vi "main_VI_one.vi"() -> ()   [LabVIEW 2019]
uses:
  <vilib>/myRIO/Instrument Drivers/Onboard IO/UART/typedef/VISA Configuration.ctl
  <vilib>/Platform/TimedLoop/XDataNode/timing_clust.ctl
  <vilib>/Platform/TimedLoop/XDataNode/nitl_modes.ctl
  <vilib>/Platform/TimedLoop/XDataNode/wakeup.ctl
  <vilib>/Instr/_visa.llb/VISA Configure Serial Port (Instr).vi
  <vilib>/FPGAPlugInAG/myRIO-1900/niLvFpga_Open_myRIO-1900.vi
  <vilib>/rvi/interface/common/dynamic/niFpgaDynamicAddResources.vi
  <vilib>/Utility/error.llb/Error Cluster From Error Code.vi
  <vilib>/rvi/errors/niLvFpgaAdjustHostInterfaceError.vi
  <vilib>/FPGAPlugInAG/Dynamic/niLvFpga_Close_Dynamic.vi
  <vilib>/rvi/interface/nirviOpenFPGA/nirviOpenFPGA.xnode
  FPGA Bitfiles/imuwired_FPGATarget_FPGAFSR_4dEayfvYof8.lvbitx
  <vilib>/Platform/TimedLoop/XDataNode/XDataNode.xnode
  <vilib>/rvi/interface/nirviReadWriteControl/nirviReadWriteControl.xnode
  <vilib>/rvi/interface/nirviCloseFPGA/nirviCloseFPGA.xnode
  <vilib>/Platform/TimedLoop/XDataNode/XDNodeRunTimeDep.lvlib
  <vilib>/myRIO/Instrument Drivers/Onboard IO/UART/UART.lvlib
  NiFpgaLv.dll
  <vilib>/rvi/interface/Simulation/niFpgaSimulationCallBeginRW.vi
panel:
  out "element out 2":dbl
  out "element out":u16
  out "# elements 2":u32
  out "# elements":u32
  out "timed out?":bool
  in  "file no.":u32
  in  "stop":bool
  in  "error in (no error)":errorcluster
  out "error out":errorcluster
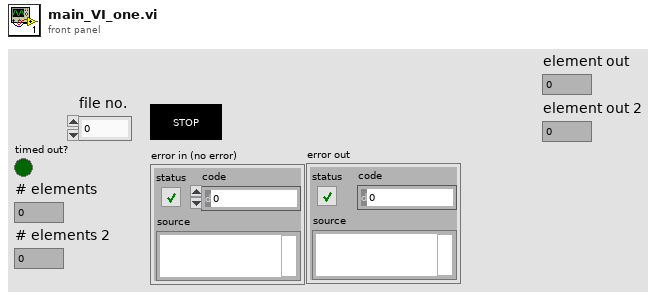
[diagram p1: front panel]
types:
  T1 = enum16{"open", "replace", "create", "open or create", "replace or create", "replace or create with confirmation"}
  T2 = cluster{"read mode":enum16{"polling", "blocking"}, "write mode":enum16{"polling", "blocking"}}
  T3 = typedef "UART.lvlib/VISA Configuration.ctl" = cluster{"baud rate (9600)":u32, "data bits (8)":u16, "parity (0:none)":enum16{"None", "Odd", "Even", "Mark", "Space"}, "stop bits (10: 1 bit)":u16, "flow control (0:none)":u16, "termination char\n(0xA = '\\n' = LF) ":u8, "Enable Termination\nChar (T)":bool, "timeout (10sec)":u32}
  T4 = typedef "XDNodeRunTimeDep.lvlib/timing_clust.ctl" = cluster{"Expected End [f-1]":u64, "Actual End [f-1]":u64, "Finished Late? [f-1]":bool, "Expected End [i-1]":u64, "Actual End [i-1]":u64, "Finished Late? [i-1]":bool, "Expected Start [i]":u64, "Actual Start [i]":u64, "Expected Start [f]":u64, "Actual Start [f]":u64, "Source Name":string, "Structure Name":string, "Period":i64, "Deadline":i64, "Offset":i64, "Start":i64, "Priority":i32, "Timeout":i32, "Mode":T5, "Wakeup Reason":T6, "Error":errorcluster, "Source Type":string, "Secondary Source Type":string, "Global End Time":u64, "Global Start Time":u64, "Frame Duration":u64, "Iteration Duration":u64, "Assigned CPU":i32, "I/O Scan Engine Mode":u32}
  T5 = typedef "XDNodeRunTimeDep.lvlib/nitl_modes.ctl" = enum32{"No Change", "Process missed periods, maintain original phase", "Discard missed periods, maintain original phase", "Process missed periods, ignore original phase", "Discard missed periods, ignore original phase"}
  T6 = typedef "XDNodeRunTimeDep.lvlib/wakeup.ctl" = enum32{"Normal", "Aborted", "Asynchronous wakeup", "Timing source error", "Timed loop error", "Timeout"}
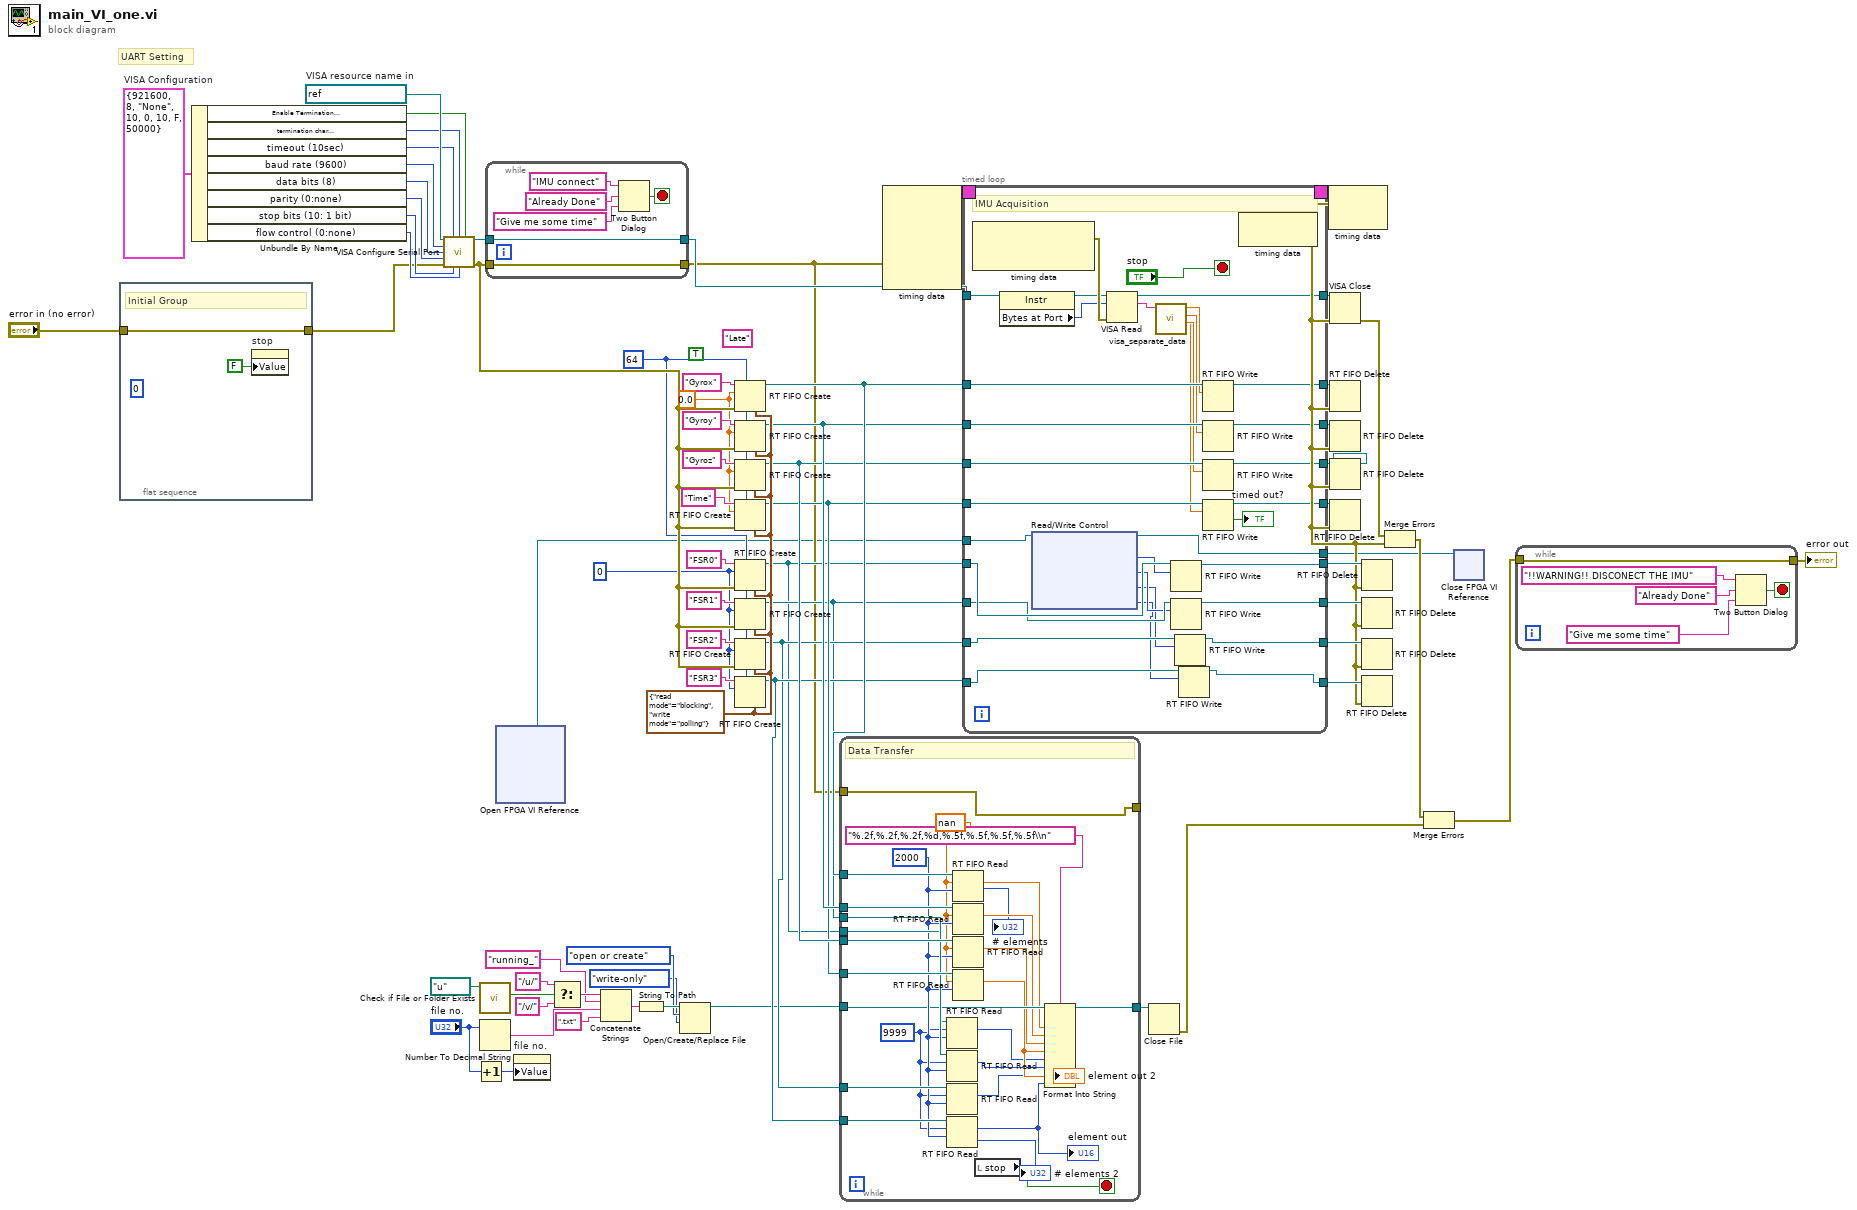
[diagram p0: block diagram]
diagram:
  w2 = u16 0
  w24 = u32 64 ("size (10)")
  (unwired) TRUE
  (unwired) "Late" ("name (unnamed)")
  w47 = T2 {"read mode"=enum."blocking", "write mode"=enum."polling"} ("r/w modes (polling,polling)")
  w25 = 0.0
  w68 = T3 {"baud rate (9600)"=921600, "data bits (8)"=8, "parity (0:none)"=enum."None", "stop bits (10: 1 bit)"=10, "flow control (0:none)"=0, "termination char\n(0xA = '\\n' = LF) "=10, "Enable Termination\nChar (T)"=FALSE, "timeout (10sec)"=50000}  # VISA Configuration
  w69 = refnum<visa-resource-name> "ASRL1::INSTR"  # VISA resource name in
  # "UART Setting"
  n1 = flat-sequence {
    tunnel: "error in (no error)" -> [w73]
    tunnel: [w73] -> w39
    frame #0 {
      (unwired) u16 0 ("On time in")
      # "Initial Group"
      n2 = property on="stop" class="Bool (strict)"("Value"=FALSE ("stop")) -> ()  [unwired: 2 in, 2 out]
    }
  }
  n3 = Unbundle By Name(w68) -> ("Enable Termination\nChar (T)"=w67:bool, "termination char\n(0xA = '\\n' = LF)"=w66:u8, "timeout (10sec)"=w65:u32, "baud rate (9600)"=w61:u32, "data bits (8)"=w62:u16, "parity (0:none)"=w63:enum16{"None", "Odd", "Even", "Mark", "Space"}, "stop bits (10: 1 bit)"=w64:u16, "flow control (0:none)"=w60:u16)
  n4 = call-poly "VISA Configure Serial Port"("VISA resource name"=w69, "timeout (10sec)"=w65, "termination char\n(0xA = '\\n' = LF)"=w66, "Enable Termination\nChar (T)"=w67, "baud rate (9600)"=w61, "data bits (8)"=w62, "parity (0:none)"=w63, "error in (no error)"=w39, "stop bits (10: 1 bit)"=w64, "flow control (0:none)"=w60) -> ("VISA resource name out"=w57:refnum<visa-resource-name>, "error out"=w49:errorcluster)  [unwired: 4 in]
  n5 = Increment(x="file no.") -> (x+1=w11:u32)
  n6 = call <vilib>:"Check if File or Folder Exists.vi"("path"=path "u:/") -> ("file or folder exists?"=w20:bool)  [unwired: 8 in, 2 out]
  n7 = Number To Decimal String(number="file no.") -> (decimal integer string=w14:string)  [unwired: 1 in]
  n8 = while {
    tunnel: [w79] -> w5
    tunnel: w49 -> [w79]
    tunnel: [w78] -> w46
    tunnel: w57 -> [w78]
    stop <- w74 stop-if-true
    n9 = Two Button Dialog(message="IMU connect", 1:"Give me some time" ("F button name (\"Cancel\")"), 2:"Already Done" ("button name (\"OK\")")) -> (T button?=w74:bool)
  }
  n10 = xnode "Open FPGA VI Reference"() -> ("FPGA VI Reference Out"=w3:refnum<k20>)  [unwired: 2 in, 1 out]
  n11 = property on="file no." class="DigNum (strict)"("Value"=w11) -> ()  [unwired: 2 in, 2 out]
  n12 = Select(t="/u/", s=w20, f="/v/") -> (s? t:f=w18:string)
  n13 = Concatenate Strings(w18, "running_" ("string"), w14, ".txt" ("string")) -> (w17:string)
  n14 = String To Path(string=w17) -> (path=w19:path)
  n15 = Open/Create/Replace File(file path (use dialog)=w19, operation (0:open)=T1."open or create", access (0:read/write)=enum16{"read/write", "read-only", "write-only"}."write-only") -> (refnum out=w9:refnum<file>)  [unwired: 3 in, 2 out]
  n16 = RT FIFO Create(0:"Gyrox" ("name (unnamed)"), 1:w25, 3:w49, 4:w24, 7:w47) -> (8:w45:refnum<k33>)  [unwired: 3 in, 2 out]
  n17 = RT FIFO Create(0:"Gyroy" ("name (unnamed)"), 1:w25, 3:w49, 4:w24, 7:w47) -> (8:w44:refnum<k33>)  [unwired: 3 in, 2 out]
  n18 = RT FIFO Create(0:"Gyroz" ("name (unnamed)"), 1:w25, 3:w49, 4:w24, 7:w47) -> (8:w43:refnum<k33>)  [unwired: 3 in, 2 out]
  n19 = RT FIFO Create(0:"Time" ("name (unnamed)"), 1:w25, 3:w49, 4:w24, 7:w47) -> (8:w42:refnum<k33>)  [unwired: 3 in, 2 out]
  n20 = RT FIFO Create(0:"FSR0" ("name (unnamed)"), 1:w2, 3:w49, 4:w24, 7:w47) -> (8:w26:refnum<k33>)  [unwired: 3 in, 2 out]
  n21 = RT FIFO Create(0:"FSR1" ("name (unnamed)"), 1:w2, 3:w49, 4:w24, 7:w47) -> (8:w27:refnum<k33>)  [unwired: 3 in, 2 out]
  n22 = RT FIFO Create(0:"FSR2" ("name (unnamed)"), 1:w2, 3:w49, 4:w24, 7:w47) -> (8:w28:refnum<k33>)  [unwired: 3 in, 2 out]
  n23 = RT FIFO Create(0:"FSR3" ("name (unnamed)"), 1:w2, 4:w24, 7:w47) -> (8:w29:refnum<k33>)  [unwired: 4 in, 2 out]
  n24 = while {
    tunnel: w45 -> [w105]
    tunnel: w44 -> [w104]
    tunnel: w43 -> [w103]
    tunnel: w42 -> [w102]
    tunnel: w29 -> [w101]
    tunnel: w28 -> [w100]
    tunnel: w27 -> [w99]
    tunnel: w26 -> [w98]
    tunnel: w9 -> [w94]
    tunnel: [w84] -> w8
    tunnel: [w95] -> _
    tunnel: w5 -> [w95]
    stop <- w97 stop-if-true
    w80 = u16 9999 ("element")
    w96 = 2000 ("timeout in ms (0)")
    w81 = nan
    # "Data Transfer"
    n25 = RT FIFO Read(0:w98, 1:w80, 2:w96) -> (9:w88:u16)  [unwired: 1 in, 4 out]
    n26 = RT FIFO Read(0:w99, 1:w80, 2:w96) -> (9:w87:u16)  [unwired: 1 in, 4 out]
    n27 = RT FIFO Read(0:w100, 1:w80, 2:w96) -> (9:w86:u16)  [unwired: 1 in, 4 out]
    n28 = RT FIFO Read(0:w101, 1:w80, 2:w96) -> (7:→"# elements 2":u32, 9:w85:u16)  [unwired: 1 in, 3 out]
    "element out" <- w85
    n29 = RT FIFO Read(0:w105, 1:w81, 2:w96) -> (7:→"# elements":u32, 9:w92:dbl)  [unwired: 1 in, 3 out]
    n30 = RT FIFO Read(0:w104, 1:w81, 2:w96) -> (9:w91:dbl)  [unwired: 1 in, 4 out]
    n31 = RT FIFO Read(0:w103, 1:w81, 2:w96) -> (9:w90:dbl)  [unwired: 1 in, 4 out]
    n32 = RT FIFO Read(0:w102, 1:w81, 2:w96) -> (9:w89:dbl)  [unwired: 1 in, 4 out]
    "element out 2" <- w89
    n33 = local read "stop"() -> (w97:bool)
    n34 = Format Into String(format string="%.2f,%.2f,%.2f,%d,%.5f,%.5f,%.5f,%.5f\\n", initial string=w94, w92, w91, w90, w89, w88, w87, w86, w85) -> (resulting string=w84:refnum<file>)  [unwired: 1 in, 1 out]
  }
  n35 = node-c288(w5) -> (w71:T4)  [unwired: 4 in]
  n36 = timed-loop {
    timing: w71 -> [_]
    timing-out: [_] -> w70
    tunnel: w46 -> [w123]
    tunnel: [w139] -> w59
    tunnel: w29 -> [w116]
    tunnel: [w115] -> w31
    tunnel: w28 -> [w111]
    tunnel: [w110] -> w32
    tunnel: w27 -> [w112]
    tunnel: [w113] -> w33
    tunnel: w26 -> [w118]
    tunnel: [w117] -> w34
    tunnel: w42 -> [w129]
    tunnel: [w128] -> w36
    tunnel: w43 -> [w135]
    tunnel: [w132] -> w35
    tunnel: w44 -> [w136]
    tunnel: [w133] -> w37
    tunnel: w45 -> [w137]
    tunnel: [w134] -> w38
    tunnel: w3 -> [w119]
    tunnel: [w106] -> w1
    stop <- "stop" stop-if-true
    # "IMU Acquisition"
    n37 = node-c288() -> (w127:errorcluster)  [unwired: 1 in, 1 out]
    n38 = property class="Instr"(reference=w123) -> (reference out=w122:refnum<visa-resource-name>, "Bytes at Port"=w121:u32)  [unwired: 1 in, 1 out]
    n39 = xnode "Read/Write Control"("FPGA VI Reference In"=w119) -> ("FPGA VI Reference Out"=w106:refnum<k20>, "ConnectorA/AI0"=w114:u16, "ConnectorA/AI1"=w109:u16, "ConnectorA/AI2"=w108:u16, "ConnectorA/AI3"=w107:u16)  [unwired: 1 in, 1 out]
    n40 = VISA Read(VISA resource name=w122, byte count=w121, error in (no error)=w127) -> (VISA resource name out=w139:refnum<visa-resource-name>, read buffer=w138:string)  [unwired: 2 out]
    n41 = call "visa_separate_data.vi"("Input string"=w138) -> ("Time"=w124:dbl, "Gyro_z"=w130:dbl, "Gyro_y"=w131:dbl, "Gyro_x"=w125:dbl)  [unwired: 7 in]
    n42 = RT FIFO Write(0:w118, 1:w114) -> (8:w117:refnum<k33>)  [unwired: 3 in, 3 out]
    n43 = RT FIFO Write(0:w112, 1:w109) -> (8:w113:refnum<k33>)  [unwired: 3 in, 3 out]
    n44 = RT FIFO Write(0:w111, 1:w108) -> (8:w110:refnum<k33>)  [unwired: 3 in, 3 out]
    n45 = RT FIFO Write(0:w116, 1:w107) -> (8:w115:refnum<k33>)  [unwired: 3 in, 3 out]
    n46 = RT FIFO Write(0:w137, 1:w125) -> (8:w134:refnum<k33>)  [unwired: 3 in, 3 out]
    n47 = RT FIFO Write(0:w136, 1:w131) -> (8:w133:refnum<k33>)  [unwired: 3 in, 3 out]
    n48 = RT FIFO Write(0:w135, 1:w130) -> (8:w132:refnum<k33>)  [unwired: 3 in, 3 out]
    n49 = RT FIFO Write(0:w129, 1:w124) -> (8:w128:refnum<k33>, 10:→"timed out?":bool)  [unwired: 3 in, 2 out]
    n50 = node-c288() -> ()  [unwired: 1 in, 1 out]
  }
  n51 = Close File(refnum=w8) -> (error out=w4:errorcluster)  [unwired: 1 in, 1 out]
  n52 = node-c288(w70) -> (w30:errorcluster)
  n53 = VISA Close(VISA resource name=w59, error in (no error)=w30) -> (error out=w41:errorcluster)
  n54 = RT FIFO Delete(0:w38, 3:w30) -> ()  [unwired: 1 in, 1 out]
  n55 = RT FIFO Delete(0:w37, 3:w30) -> ()  [unwired: 1 in, 1 out]
  n56 = RT FIFO Delete(0:w35, 3:w30) -> ()  [unwired: 1 in, 1 out]
  n57 = RT FIFO Delete(0:w36, 3:w30) -> ()  [unwired: 1 in, 1 out]
  n58 = RT FIFO Delete(0:w34, 3:w30) -> ()  [unwired: 1 in, 1 out]
  n59 = RT FIFO Delete(0:w33, 3:w30) -> ()  [unwired: 1 in, 1 out]
  n60 = RT FIFO Delete(0:w32, 3:w30) -> ()  [unwired: 1 in, 1 out]
  n61 = RT FIFO Delete(0:w31, 3:w30) -> ()  [unwired: 1 in, 1 out]
  n62 = Merge Errors(w41, w30) -> (w7:errorcluster)
  n63 = Merge Errors(w7, w4) -> (w6:errorcluster)
  n64 = xnode "Close FPGA VI Reference"("FPGA VI Reference In"=w1) -> ()  [unwired: 1 in, 1 out]
  n65 = while {
    tunnel: [w147] -> w58
    tunnel: w6 -> [w147]
    stop <- w143 stop-if-true
    n66 = Two Button Dialog(message="!!WARNING!! DISCONECT THE IMU", 1:"Give me some time" ("F button name (\"Cancel\")"), 2:"Already Done" ("button name (\"OK\")")) -> (T button?=w143:bool)
  }
  "error out" <- w58
